vi "Write File.vi"(8 "error in":errorcluster, 11 "tCRD in":refnum<class "Aircraft OPCCRD.lvclass">) -> (0 "error out":errorcluster, 3 "tCRD out":refnum<class "Aircraft OPCCRD.lvclass">)   [LabVIEW 2015, in "Aircraft OPCCRD.lvclass"]
uses:
  Aircraft OPCCRD.lvclass
  Aircraft OPCCRD.lvclass/Aircraft OPCCRD.ctl
  Reusable/File IO/Class/File Observer.lvclass
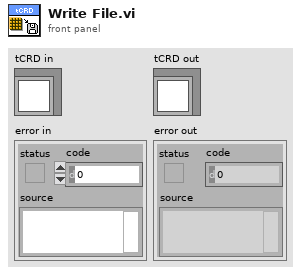
[diagram p1: front panel]
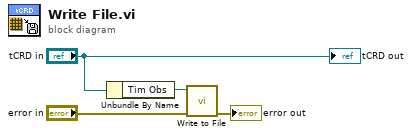
[diagram p0: block diagram]
diagram:
  n1 = Unbundle By Name("tCRD in") -> ("Tim Obs"=w4:refnum<class "Tim File Observer.lvclass">)
  n2 = call "Write to File.vi"("error in"="error in", "File Obs in"=w4) -> ("error out"=→"error out":errorcluster)  [unwired: 8 in, 1 out]
  "tCRD out" <- "tCRD in"
